vi "Bank - Race Condition.vi"() -> ()   [LabVIEW 2012]
doc: "本VI模拟银行事务，演示竞争状态。\n\n运行本VI，尝试并发事务，观察存款或取款操作丢失的情况。尝试查找并解决该问题。"
panel:
  out "余额":dbl
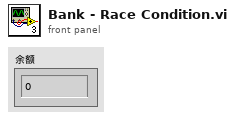
[diagram p1: front panel]
types:
  T1 = typedef "Account Info.ctl" = cluster{"银行集合点":T2, "取款队列":refnum<queue>, "存款队列":refnum<queue>}
  T2 = typedef "Rendezvous RefNum" = refnum<k1>
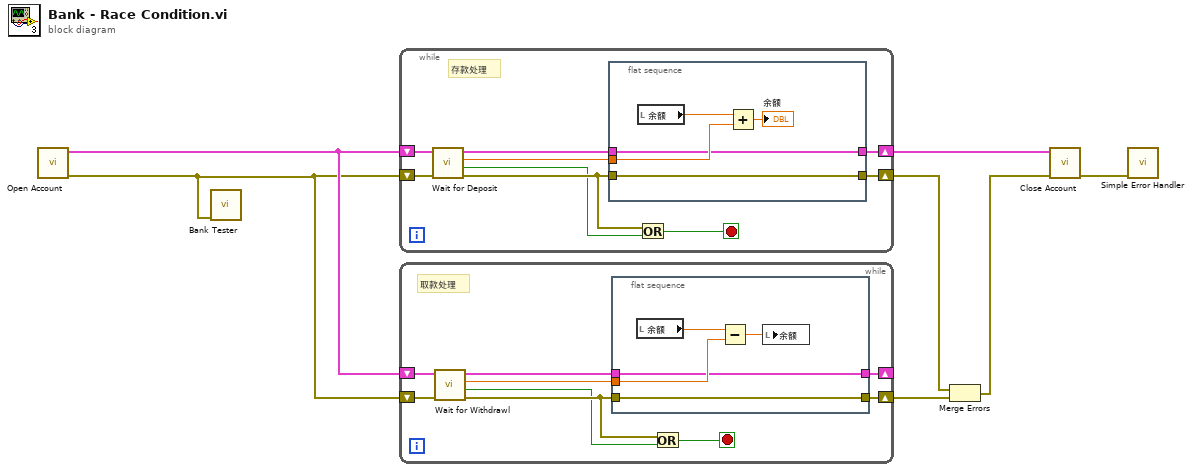
[diagram p0: block diagram]
diagram:
  n1 = call "Open Account.vi"() -> ("错误输出"=w1:errorcluster, "帐户信息"=w7:T1)  [unwired: 10 in]
  n2 = call "Bank Tester.vi"("错误输入"=w1) -> ()  [unwired: 10 in, 1 out]
  n3 = while {
    shift-right: [w12] -> w4
    shift-left: w7 -> [w15]
    shift-right: [w11] -> w6
    shift-left: w1 -> [w14]
    stop <- w8 stop-if-true
    # "存款处理"
    n4 = call "Wait for Deposit.vi"("错误输入"=w14, "帐户信息"=w15) -> ("错误输出"=w10:errorcluster, "停止？"=w9:bool, "存款额"=w16:dbl, "帐户信息输出"=w13:T1)  [unwired: 6 in]
    n5 = flat-sequence {
      tunnel: w16 -> [w21]
      tunnel: [w18] -> w12
      tunnel: w13 -> [w18]
      tunnel: w10 -> [w17]
      tunnel: [w17] -> w11
      frame #0 {
        n6 = local read "余额"() -> (w19:dbl)
        n7 = Add ("加")(x=w19, y=w21) -> (x+y=→"余额":dbl)
      }
    }
    n8 = Or ("或")(x=w10, y=w9) -> (x .or. y?=w8:bool)
  }
  n9 = while {
    shift-right: [w26] -> _
    shift-left: w7 -> [w29]
    shift-right: [w25] -> w5
    shift-left: w1 -> [w28]
    stop <- w22 stop-if-true
    # "取款处理"
    n10 = call "Wait for Withdrawl.vi"("错误输入"=w28, "帐户信息"=w29) -> ("错误输出"=w24:errorcluster, "停止？"=w23:bool, "取款额"=w30:dbl, "帐户信息输出"=w27:T1)  [unwired: 6 in]
    n11 = flat-sequence {
      tunnel: w30 -> [w33]
      tunnel: w27 -> [w32]
      tunnel: w24 -> [w31]
      tunnel: [w32] -> w26
      tunnel: [w31] -> w25
      frame #0 {
        n12 = local read "余额"() -> (w34:dbl)
        n13 = Subtract ("减")(x=w34, y=w33) -> (x-y=w35:dbl)
        n14 = local write "余额"(w35) -> ()
      }
    }
    n15 = Or ("或")(x=w24, y=w23) -> (x .or. y?=w22:bool)
  }
  n16 = Merge Errors ("合并错误")(w6, w5) -> (w2:errorcluster)
  n17 = call "Close Account.vi"("错误输入"=w2, "帐户信息"=w4) -> ("错误输出"=w3:errorcluster)  [unwired: 9 in]
  n18 = call <vilib>:"Simple Error Handler.vi"("error in (no error)"=w3) -> ()  [unwired: 4 in, 5 out]
